vi "Simple Put Multiple Files.vi"(0 "host uri":string, 1 "username":string, 2 "password":string, 5 "file specifications":T1(array[cluster]), 11 "error in (no error)":errorcluster) -> (15 "error out":errorcluster)   [LabVIEW 2017, in "NI_WebDAV.lvlib"]
doc: "Uploads a file or multiple files to a remote WebDAV server or target. You must manually select the polymorphic instance you want to use."
uses:
  <vilib>/WebDAVClient/NI_WebDAV.lvlib
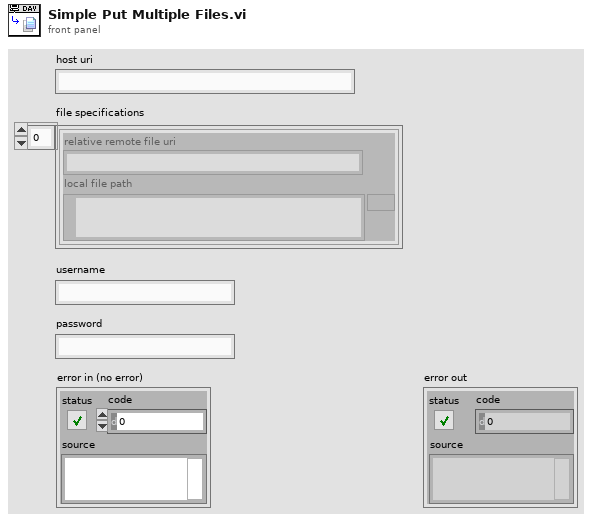
[diagram p1: front panel]
types:
  T1 = cluster{"relative remote file uri":string, "local file path":path}[]
  T2 = typedef "NI_WebDAV.lvlib/SessionHandle.ctl" = refnum<k1>
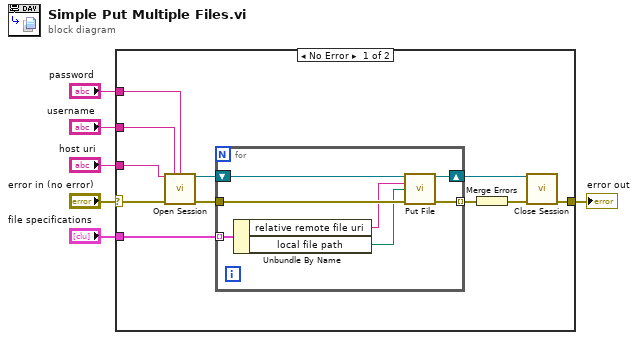
[diagram p0: block diagram]
diagram:
  n1 = case shown="No Error" "error in (no error)" {
    selector: "error in (no error)" -> [w17 w25]
    tunnel: "file specifications" -> [w12 _]
    tunnel: "host uri" -> [w8 _]
    tunnel: "username" -> [w16 _]
    tunnel: "password" -> [w15 _]
    tunnel: [w9 w25] -> w1
    frame No Error {
      n2 = call <vilib>:"Open Session.vi"("host uri prefix"=w8, "username"=w16, "password"=w15, "error in (no error)"=w17) -> ("session handle out"=w13:T2, "error out"=w14:errorcluster)  [unwired: 10 in]
      n3 = for {
        shift-right: [w20] -> w10
        shift-left: w13 -> [w22]
        tunnel: w14 -> [w23]
        tunnel: w12 -> [w24] mode=indexing
        tunnel: [w19] -> w7 mode=indexing
        n4 = Unbundle By Name(w24) -> ("relative remote file uri"=w21:string, "local file path"=w18:path)
        n5 = call <vilib>:"Put File.vi"("session handle"=w22, "relative uri"=w21, "local file path"=w18, "error in (no error)"=w23) -> ("session handle out"=w20:T2, "error out"=w19:errorcluster)  [unwired: 9 in, 1 out]
      }
      n6 = Merge Errors(w7) -> (w11:errorcluster)
      n7 = call <vilib>:"Close Session.vi"("session handle"=w10, "error in (no error)"=w11) -> ("error out"=w9:errorcluster)  [unwired: 13 in]
    }
    frame Error {
    }
  }
  "error out" <- w1
